vi "Create Mask By Index.vi"(10 "Color Palette Index (0)":u8, 11 "Image":T1) -> (3 "Masked Image":T1)   [LabVIEW 2020, in "G-Image.lvlib"]
doc: "Creates an image mask based on the index into the image's color palette table. Applies to 8-bit images only.\n\nSimilar to LabVIEW's <b>Create Mask.vi</b> and <b>Create Mask By Alpha.vi</b>."
uses:
  G-Image.lvlib
  <vilib>/picture/picture.llb/imagedata.ctl
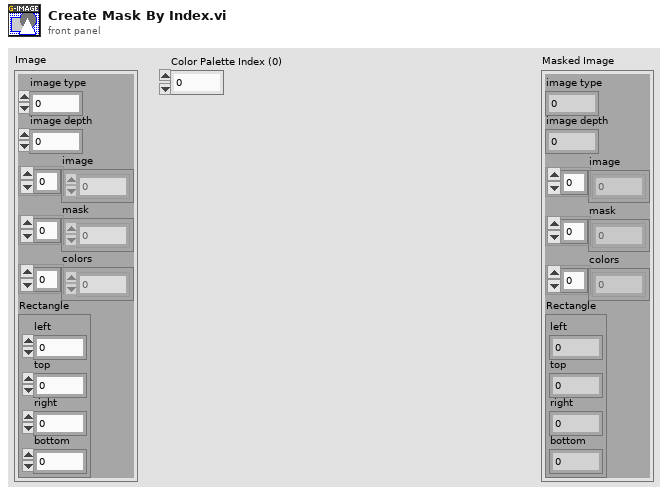
[diagram p1: front panel]
types:
  T1 = typedef "imagedata.ctl" = cluster{"image type":i32, "image depth":i32, "image":u8[], "mask":u8[], "colors":u32[], "Rectangle":cluster{"left":i16, "top":i16, "right":i16, "bottom":i16}}
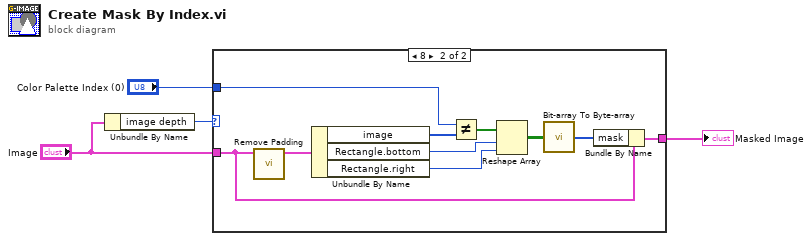
[diagram p0: block diagram]
diagram:
  n1 = Unbundle By Name("Image") -> ("image depth"=w3:i32)
  n2 = case shown="8" w3 {
    tunnel: "Image" -> [w5 w8]
    tunnel: [w5 w6] -> w2
    tunnel: "Color Palette Index (0)" -> [_ w9]
    frame Default {
    }
    frame 8 {
      n3 = call "Remove Padding.vi"("Image"=w8) -> ("Image Out"=w10:T1)  [unwired: 9 in, 1 out]
      n4 = Unbundle By Name(w10) -> ("image"=w15:u8[], "Rectangle.bottom"=w12:i16, "Rectangle.right"=w11:i16)
      n5 = Not Equal?(x=w9, y=w15) -> (x != y?=w14:bool[])
      n6 = Reshape Array(w14, w12, w11) -> (w13:bool[][])
      n7 = call <vilib>:"Bit-array To Byte-array.vi"("bit array"=w13) -> ("byte array"=w7:u8[])
      n8 = Bundle By Name(cluster=w8, "mask"=w7) -> (w6:T1)
    }
  }
  "Masked Image" <- w2
